vi "RT Loop - Analyze Acceleration_V2_no_kistler.vi"(7 "testing":bool, 8 "error in (no error)":errorcluster, 9 "Acceleration RT FIFO In":T1, 10 "FPGA VI Reference Out 2":refnum<k20>, 11 "Message Queue":refnum<queue>) -> (1 "Acceleration RT FIFO Out":T1)   [LabVIEW 2017]
doc: "Read and analyze acceleration waveform data from FPGA via DMA FIFO. If the acceleration is over the limit, then send the acceleration waveform data to the Log Data Loop."
uses:
  UI Error Handlers/support/Message Queue/Message Cluster.ctl
  controls/Acceleration RT FIFO Reference.ctl
  data_sav.ctl
  Control 1.ctl
  Globals/Global - All RT Loop Stop.vi
  Globals/Global - Configuration Options.vi
  <vilib>/Utility/error.llb/Error Cluster From Error Code.vi
  <vilib>/rvi/errors/niLvFpgaAdjustHostInterfaceError.vi
  <vilib>/rvi/interface/nirviMethod/nirviMethod.xnode
  <vilib>/FPGAPlugInAG/Dynamic/niLvFpga_ReadFifo_Dynamic.vi
  <vilib>/rvi/errors/niLvFpgaMergeErrorWithErrorCode.vi
  UI Error Handlers/support/Logging/Logging.lvlib
  UI Error Handlers/support/Message Queue/Message Queue.lvlib
panel:
  out "Free Physical Memory or Largest Contiguous Memory (bytes)":i64(graph)
  out "error out":errorcluster
  out "x-y":u32
  out "G1 status":cluster{"G1 trigger":bool}
  out "G1 status.G1 trigger":bool
  out "sta":bool
  out "logical OR":bool
  in  "Data Rate (Hz)":dbl
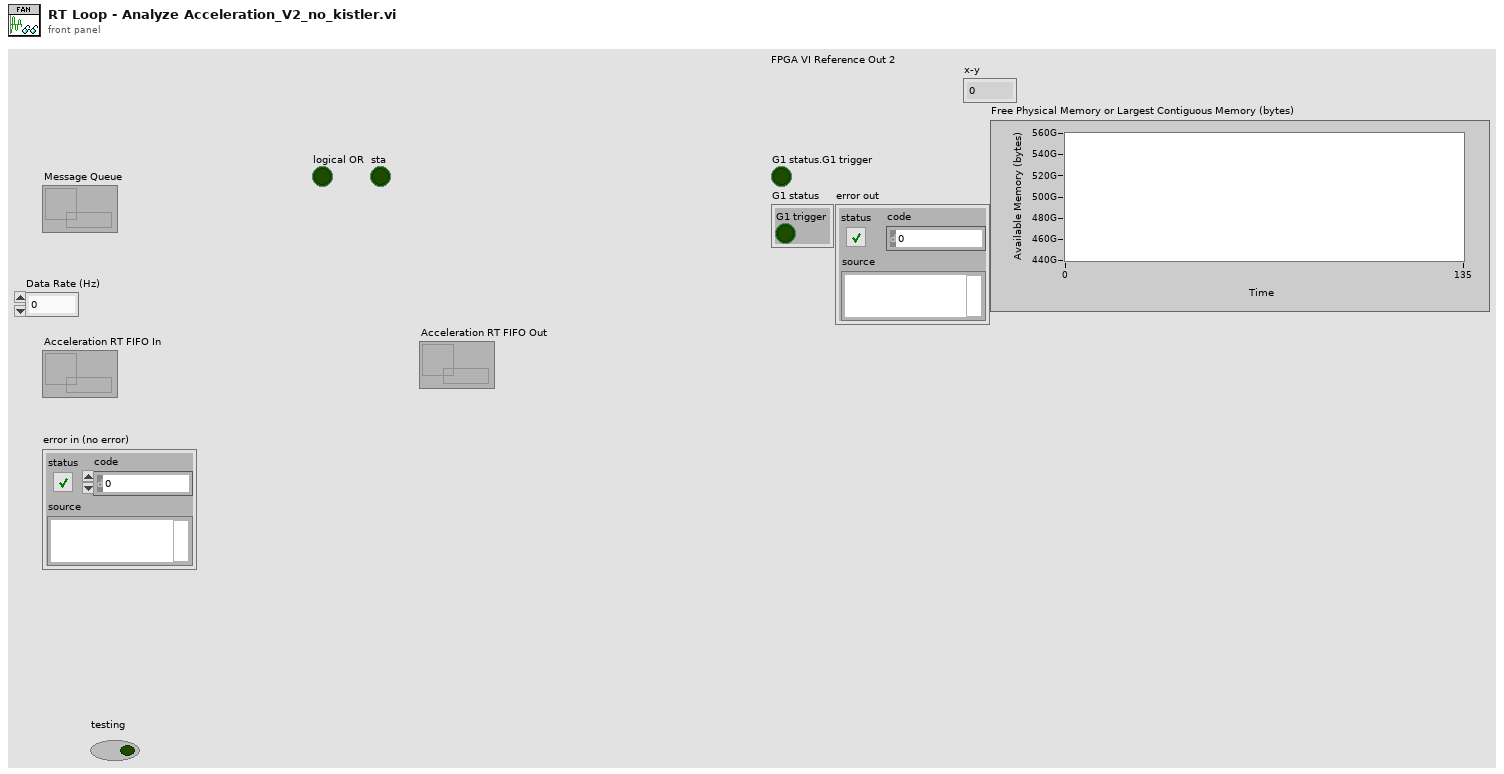
[diagram p1: front panel]
types:
  T1 = typedef "Acceleration RT FIFO Reference.ctl" = refnum<k33>
  T2 = typedef "data_sav.ctl" = cluster{"Log File out 2":refnum<k34>, "Array":T3[]}
  T3 = typedef "Control 1.ctl" = waveform(dbl)
  T4 = cluster{"Tool data":cluster{"Number of teeth":sgl}, "Cutting data":cluster{"rpm":sgl}, "Limits":cluster{"Magnitude threshold":sgl, "Tolerance":sgl}, "G1 status":cluster{"G1 trigger":bool}}
  T5 = cluster{"Log File out":refnum<k34>, waveform(dbl)[]}
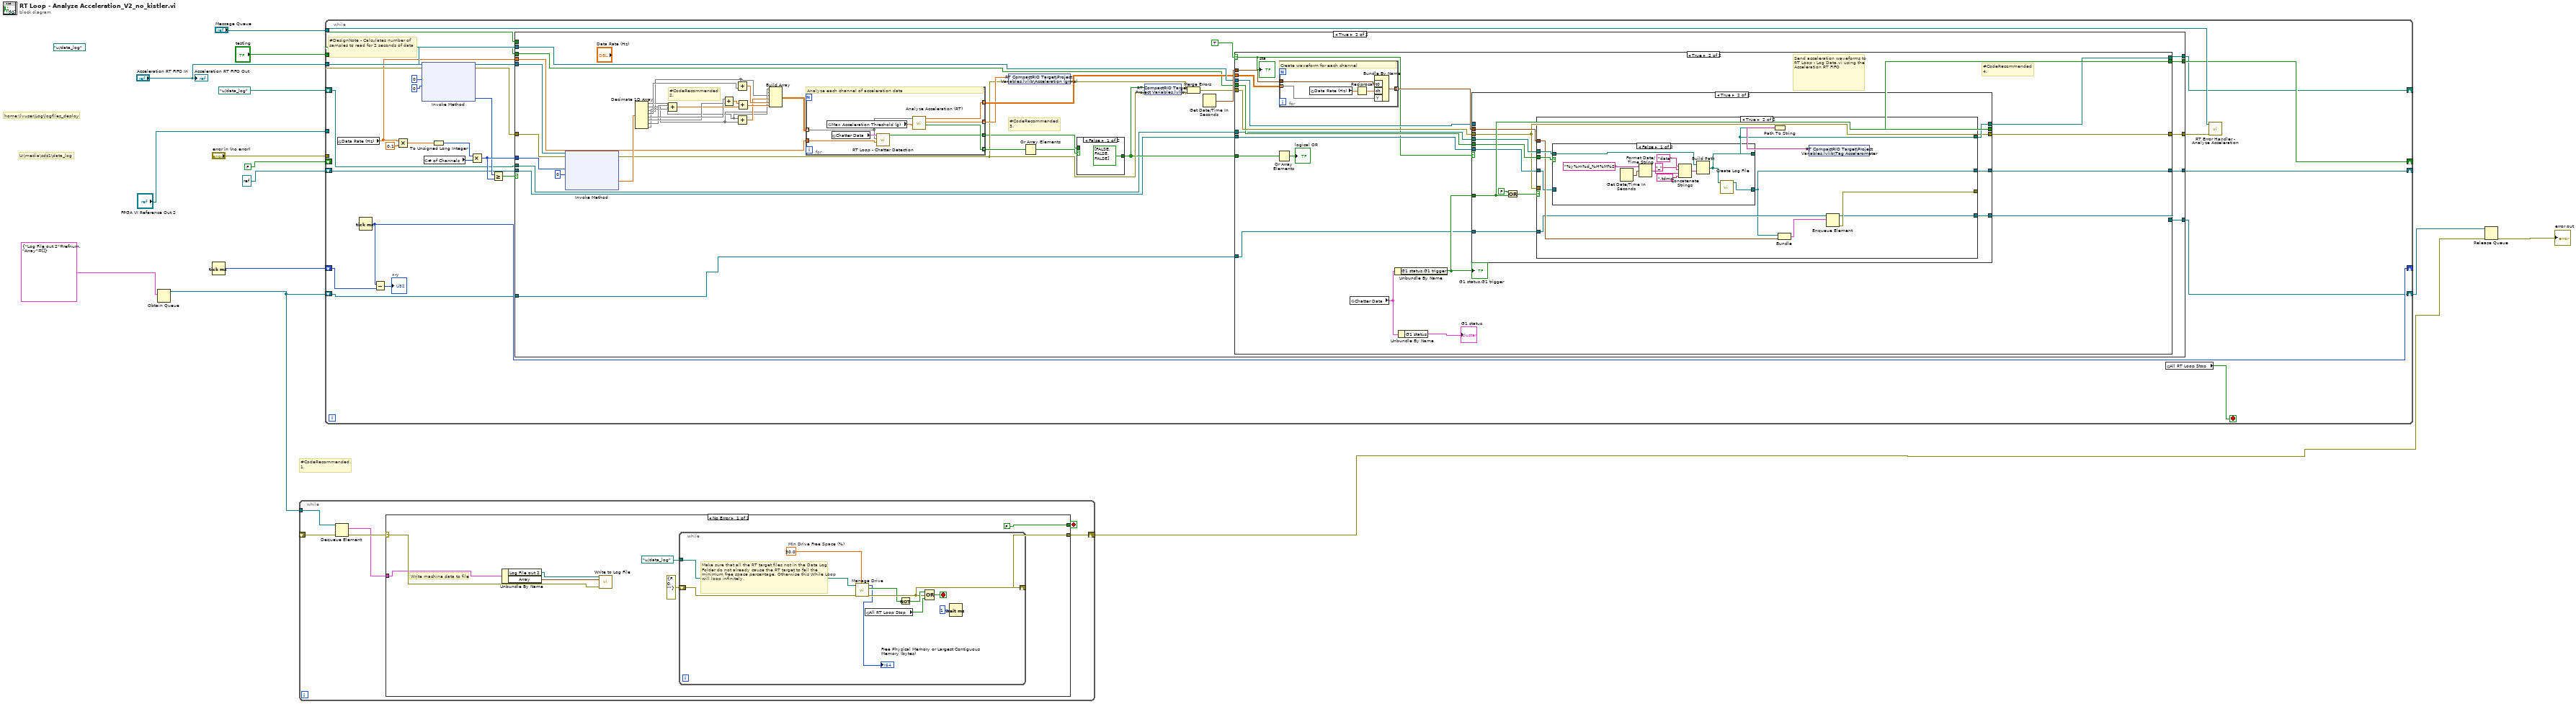
[diagram p0: block diagram]
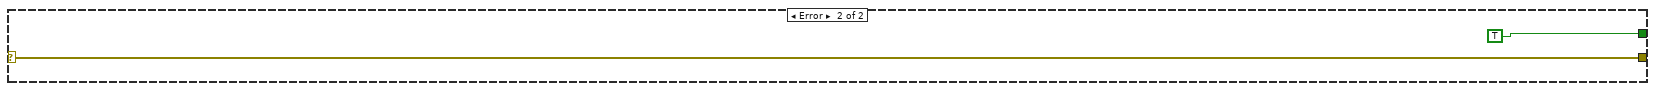
[diagram p2: hidden frame]
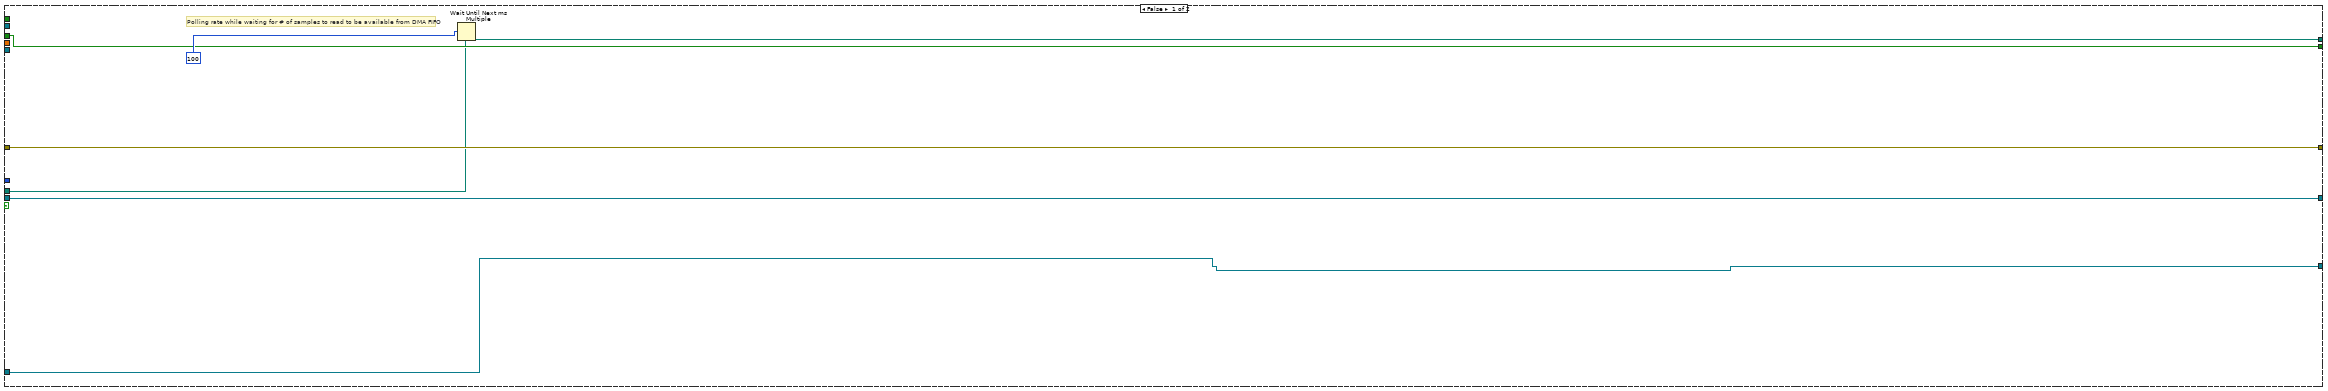
[diagram p3: hidden frame]
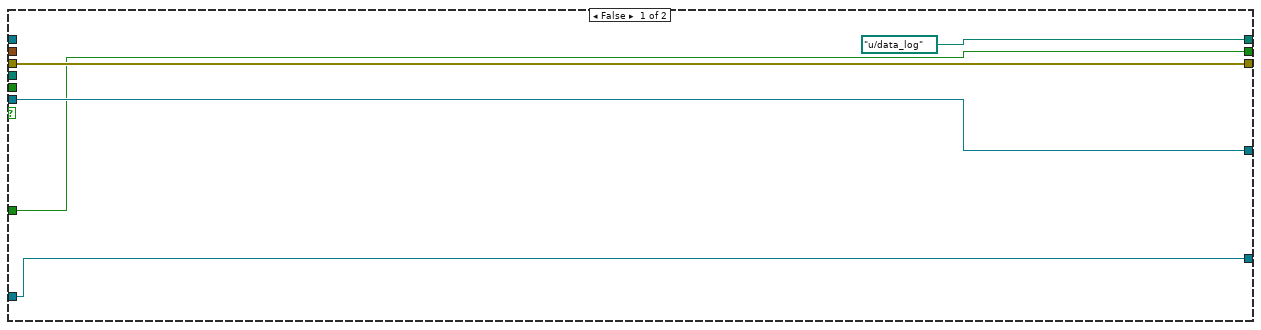
[diagram p6: hidden frame]
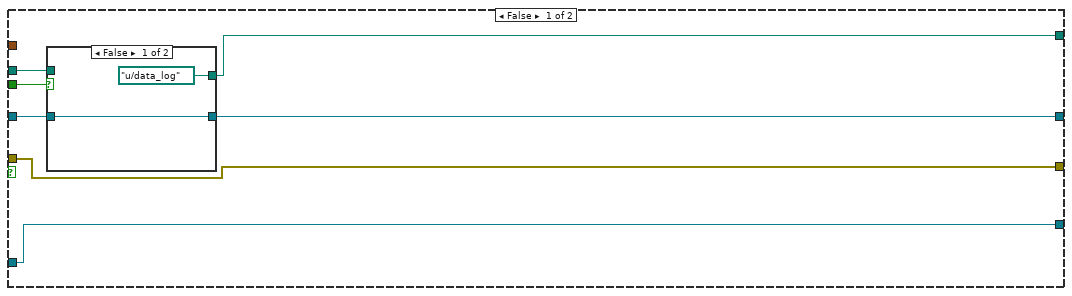
[diagram p7: hidden frame]
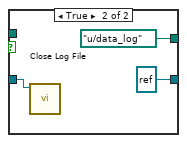
[diagram p8: hidden frame]
diagram:
  (unwired) path "u:/data_log" ("AVI Path")
  # "U:\\media\\sdc1\\data_log"
  # "home:\\lvuser\\Log\\logfiles_deploy"
  # "#CodeRecommended\n1."
  n1 = Obtain Queue(element data type=T2 {"Log File out 2"=refnum, "Array"=[]}) -> (queue out=w4:refnum<queue>)  [unwired: 4 in, 2 out]
  n2 = Tick Count (ms)() -> (millisecond timer value=w7:u32)
  n3 = while {
    tunnel: w4 -> [w20]
    shift-right: [w16] -> w2
    shift-left: _ -> [w19]
    stop <- w17 stop-if-true
    n4 = Dequeue Element(queue=w20, error in (no error)=w19) -> (element=w15:T2, error out=w18:errorcluster)  [unwired: 1 in, 2 out]
    n5 = case shown="No Error" w18 {
      selector: w18 -> [w25 w39]
      tunnel: [FALSE TRUE] -> w17
      tunnel: [w26 w39] -> w16
      tunnel: w15 -> [w24 _]
      frame No Error {
        # "Write machine data to file"
        n6 = Unbundle By Name(w24) -> ("Log File out 2"=w23:refnum<k34>, "Array"=w22:T3[])
        n7 = call "Write to Log File.vi"("error in (no error)"=w25, "Array of Waveforms"=w22, "Log File in"=w23) -> ()  [unwired: 7 in, 2 out]
        n8 = while {
          shift-right: [w33] -> w26
          shift-left: errorcluster {"status"=FALSE, "code"=0, "source"=""} ("error out") -> [w34]
          tunnel: path "u:/data_log" ("AVI Path") -> [w31]
          stop <- w38 stop-if-true
          w32 = 30.0  # Min Drive Free Space (%)
          # "Make sure that all the RT target files not in the Data Log Folder do not already cause the RT target to fail the minimum free space percentage. Otherwise this While Loop will loop infinitely."
          n9 = call "Manage Drive.vi"("Min Drive Free Space (%)"=w32, "error in"=w34, "Data Folder"=w31) -> ("error out"=w33:errorcluster, "Drive Space Below Limit"=w30:bool, "size (bytes)"=→"Free Physical Memory or Largest Contiguous Memory (bytes)":i64)  [unwired: 6 in]
          n10 = global read "Global - All RT Loop Stop.vi" "All RT Loop Stop"() -> (w35:bool)
          n11 = Not(x=w30) -> (.not. x?=w37:bool)
          n12 = Compound Arithmetic op=OR(w37, w33, w35) -> (w38:bool)
          n13 = Wait (ms)(milliseconds to wait=u32 1) -> ()  [unwired: 1 out]
        }
      }
      frame Error {
      }
    }
  }
  n14 = while {
    tunnel: "FPGA VI Reference Out 2" -> [w70]
    tunnel: "error in (no error)" -> [w69]
    tunnel: "Message Queue" -> [w62]
    tunnel: "Acceleration RT FIFO In" -> [w60]
    tunnel: "testing" -> [w52]
    shift-right: [w49] -> _
    shift-left: path "u:/data_log" ("AVI Path") -> [w48]
    shift-right: [w51] -> _
    shift-left: FALSE -> [w50]
    shift-right: [w47] -> _
    shift-left: refnum<k34> refnum ("Log File out") -> [w46]
    shift-right: [w44] -> _
    shift-left: w7 -> [w45]
    shift-right: [w41] -> w3
    shift-left: w4 -> [w42]
    stop <- w63 stop-if-true
    # "#DesignNote - Calculates number of samples to read for 2 seconds of data"
    n15 = global read "Global - Configuration Options.vi" "Data Rate (Hz)"() -> (w54:dbl)
    n16 = Tick Count (ms)() -> (millisecond timer value=w44:u32)
    n17 = Subtract(x=w44, y=w45) -> (x-y=→"x-y":u32)
    n18 = Multiply(x=w54, y=0.1) -> (x*y=w58:dbl)
    n19 = xnode "Invoke Method"("FPGA VI Reference In"=w70, "error in"=w69, "Number of Elements"=u32 0, "Timeout (ms)"=0) -> ("FPGA VI Reference Out"=w66:refnum<k20>, "error out"=w65:errorcluster, "Elements Remaining"=w53:u32)  [unwired: 1 out]
    n20 = global read "Global - Configuration Options.vi" "# of Channels"() -> (w55:u32)
    n21 = To Unsigned Long Integer(number=w58) -> (unsigned 32bit integer=w57:u32)
    n22 = Multiply(x=w57, y=w55) -> (x*y=w56:u32)
    n23 = Greater Or Equal?(x=w53, y=w56) -> (x >= y?=w64:bool)
    n24 = case shown="True" w64 {
      tunnel: w66 -> [_ w118]
      tunnel: w65 -> [w76 w117]
      tunnel: [w76 w113] -> w61
      tunnel: w56 -> [_ w116]
      tunnel: w60 -> [_ w111]
      tunnel: w54 -> [_ w107]
      tunnel: w52 -> [_ _]
      tunnel: [w74 w99] -> w51
      tunnel: w50 -> [w74 w98]
      tunnel: [w73 w97] -> w49
      tunnel: w48 -> [w73 w96]
      tunnel: [w72 w95] -> w47
      tunnel: w46 -> [w72 w94]
      tunnel: w42 -> [w71 w82]
      tunnel: [w71 w81] -> w41
      frame False {
        # "Polling rate while waiting for # of samples to read to be available from DMA FIFO"
        n25 = Wait Until Next ms Multiple(millisecond multiple=u32 100) -> ()  [unwired: 1 out]
      }
      frame True {
        # "#CodeRecommended\n3."
        # "#CodeRecommended\n2."
        n26 = xnode "Invoke Method"("FPGA VI Reference In"=w118, "error in"=w117, "Number of Elements"=w116, "Timeout (ms)"=0) -> ("error out"=w106:errorcluster, "Data"=w110:sgl[])  [unwired: 2 out]
        n27 = Decimate 1D Array(w110) -> (w79:sgl[], w78:sgl[], w77:sgl[], w91:sgl[], w90:sgl[], w89:sgl[], w88:sgl[], w87:sgl[])
        n28 = Add(x=w88, y=w87) -> (x+y=w85:sgl[])
        n29 = Add(x=w90, y=w89) -> (x+y=w86:sgl[])
        n30 = Add(x=w77, y=w91) -> (x+y=w83:sgl[])
        n31 = Add(x=w79, y=w78) -> (x+y=w80:sgl[])
        n32 = Add(x=w86, y=w85) -> (x+y=w84:sgl[])
        n33 = Build Array(w79, w78, w77, w80, w83, w84) -> (w92:sgl[][])
        n34 = for {
          tunnel: [w128] -> w112 mode=indexing
          tunnel: [w127] -> w109 mode=indexing
          tunnel: [w126] -> w108 mode=indexing
          tunnel: w107 -> [w124]
          tunnel: [w123] -> w101 mode=indexing
          tunnel: w92 -> [w121] mode=indexing
          # "Analyze each channel of acceleration data"
          n35 = global read "Global - Configuration Options.vi" "Max Acceleration Threshold (g)"() -> (w125:sgl)
          n36 = global read "Global - Configuration Options.vi" "Chatter Data"() -> (w122:T4)
          n37 = call "RT Loop - Chatter Detection.vi"("Data Rate (Hz)"=w124, "Acceleration Waveform (SGL)"=w121, "Chatter Data"=w122) -> ("Chatter?"=w123:bool)  [unwired: 8 in]
          n38 = call "Analyze Acceleration (RT).vi"("Max Instantaneous Acceleration (g)"=w125, "Acceleration Waveform (SGL)"=w121) -> ("Over Limit?"=w128:bool, "Acceleration (grms)"=w126:dbl, "Acceleration Waveform (DBL)"=w127:dbl[])  [unwired: 7 in]
        }
        n39 = shared-variable "RT CompactRIO Target\\Project Variables.lvlib\\Acceleration (grms)"(w108, error in=w106) -> (error out=w104:errorcluster)
        n40 = Or Array Elements(Boolean array=w112) -> (logical OR=w102:bool)
        n41 = case shown="False" w102 {
          tunnel: w101 -> [_ w120]
          tunnel: [bool[] [FALSE, FALSE, FALSE] ("Chatter?") w120] -> w100
          frame False {
          }
          frame True {
          }
        }
        n42 = shared-variable "RT CompactRIO Target\\Project Variables.lvlib\\Chatter?"(w100, error in=w106) -> (error out=w105:errorcluster)
        n43 = Merge Errors(w104, w105) -> (w103:errorcluster)
        n44 = Get Date/Time In Seconds() -> (seconds since 1Jan1904=w114:timestamp)
        n45 = case shown="True" TRUE {
          selector: TRUE -> [_ w134]
          tunnel: w114 -> [_ w153]
          tunnel: w103 -> [w133 w152]
          tunnel: [w133 w137] -> w113
          tunnel: w111 -> [_ w150]
          tunnel: w109 -> [_ w149]
          tunnel: w100 -> [_ w147]
          tunnel: [w132 w144] -> w99
          tunnel: w98 -> [w132 w143]
          tunnel: [w131 w142] -> w97
          tunnel: w96 -> [w131 w138]
          tunnel: [w130 w141] -> w95
          tunnel: w94 -> [w130 w140]
          tunnel: w82 -> [w129 w136]
          tunnel: [w129 w135] -> w81
          frame False {
          }
          frame True {
            # "#CodeRecommended\n4."
            # "Send acceleration waveforms to RT Loop - Log Data.vi using the Acceleration RT FIFO"
            n46 = Or Array Elements(Boolean array=w147) -> (logical OR=→"logical OR":bool)
            n47 = for {
              tunnel: w149 -> [w210] mode=indexing
              tunnel: w153 -> [w209]
              tunnel: [w207] -> w151 mode=indexing
              # "Create waveform for each channel"
              n48 = global read "Global - Configuration Options.vi" "Data Rate (Hz)"() -> (w206:dbl)
              n49 = Reciprocal(x=w206) -> (1/x=w208:dbl)
              n50 = Bundle By Name("t0"=w209, "dt"=w208, "Y"=w210) -> (w207:waveform(dbl))  [unwired: 1 in]
            }
            n51 = global read "Global - Configuration Options.vi" "Chatter Data"() -> (w146:T4)
            n52 = Unbundle By Name(w146) -> ("G1 status.G1 trigger"=w139:bool)
            "G1 status.G1 trigger" <- w139
            n53 = Unbundle By Name(w146) -> ("G1 status"=→"G1 status":cluster{"G1 trigger":bool})
            n54 = case shown="True" w134 {
              tunnel: w152 -> [w158 w161]
              tunnel: w151 -> [_ w162]
              tunnel: w150 -> [_ _]
              tunnel: w139 -> [w156 w168]
              tunnel: [w156 w168] -> w144
              tunnel: w143 -> [_ w167]
              tunnel: [path "u:/data_log" ("AVI Path") w166] -> w142
              tunnel: w138 -> [_ w165]
              tunnel: [w157 w164] -> w141
              tunnel: w140 -> [w157 w163]
              tunnel: [w158 w161] -> w137
              tunnel: w136 -> [w154 w159]
              tunnel: [w154 w160] -> w135
              frame False {
              }
              frame True {
                n55 = Or(x=FALSE, y=w168) -> (x .or. y?=w170:bool)
                n56 = case shown="True" w170 {
                  tunnel: w165 -> [w174 w193]
                  tunnel: [w177 w190] -> w166
                  tunnel: w167 -> [w175 w192]
                  tunnel: w163 -> [w176 w184]
                  tunnel: w162 -> [_ w186]
                  tunnel: [w173 w183] -> w164
                  tunnel: w161 -> [w172 _]
                  tunnel: [w172 w189] -> _
                  tunnel: w159 -> [w171 w185]
                  tunnel: [w171 w188] -> w160
                  frame False {
                    n57 = case shown="False" w175 {
                      tunnel: [path "u:/data_log" ("AVI Path") path "u:/data_log" ("AVI Path")] -> w177
                      tunnel: w176 -> [w178 w181]
                      tunnel: w174 -> [_ _]
                      tunnel: [w178 refnum<k34> refnum ("Log File out")] -> w173
                      frame False {
                      }
                      frame True {
                        n58 = call "Close Log File.vi"("tdms file"=w181) -> ()  [unwired: 10 in, 1 out]
                      }
                    }
                  }
                  frame True {
                    n59 = case shown="False" w192 {
                      tunnel: w193 -> [w196 w205]
                      tunnel: [w195 w205] -> w190
                      tunnel: [w194 w204] -> w183
                      tunnel: w184 -> [_ w204]
                      frame False {
                        n60 = Get Date/Time In Seconds() -> (seconds since 1Jan1904=w199:timestamp)
                        n61 = Format Date/Time String(time format string (%c)="%y%m%d_%H%M%S", seconds (now)=w199) -> (date/time string=w202:string)  [unwired: 1 out]
                        n62 = Concatenate Strings("data" ("string"), "_" ("string"), w202, ".tdms" ("string")) -> (w197:string)
                        n63 = Build Path(base path=w196, name or relative path=w197) -> (appended path=w195:path)
                        n64 = call "Create Log File.vi"("Acceleration Exceeded Log Folder"=w195) -> ("Log File out"=w194:refnum<k34>)  [unwired: 9 in, 1 out]
                      }
                      frame True {
                      }
                    }
                    n65 = Path To String(path=w190) -> (string=w191:string)
                    n66 = Bundle("Log File out"=w183, w186) -> (w187:T5)  [unwired: 1 in]
                    n67 = shared-variable "RT CompactRIO Target\\Project Variables.lvlib\\Tag Accelerometer"(w191) -> ()  [unwired: 1 in, 1 out]
                    n68 = Enqueue Element(queue=w185, element=w187) -> (queue out=w188:refnum<queue>, error out=w189:errorcluster)  [unwired: 2 in, 1 out]
                  }
                }
              }
            }
            "sta" <- w134
          }
        }
      }
    }
    n69 = global read "Global - All RT Loop Stop.vi" "All RT Loop Stop"() -> (w63:bool)
    n70 = call "RT Error Handler - Analyze Acceleration.vi"("error in (no error)"=w61, "Message Queue"=w62) -> ()  [unwired: 9 in, 1 out]
  }
  n71 = Release Queue(queue=w3, error in (no error)=w2) -> (error out=→"error out":errorcluster)  [unwired: 1 in, 2 out]
  "Acceleration RT FIFO Out" <- "Acceleration RT FIFO In"
